vi "getParameters.vi"(8 "error in":errorcluster, 11 "Time in":refnum<class "Time.lvclass">) -> (0 "error out":errorcluster, 2 "Time.Parameters":T1, 3 "Time out":refnum<class "Time.lvclass">)   [LabVIEW 2022 SP3, in "Time.lvclass"]
uses:
  Time.lvclass
  Time.Parameters.ctl
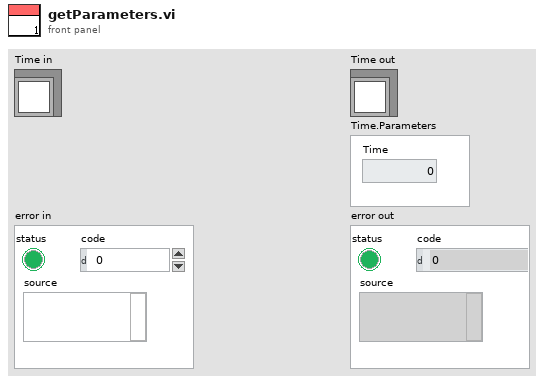
[diagram p1: front panel]
types:
  T1 = typedef "Time.lvclass/Time.Parameters.ctl" = cluster{"Time":u32}
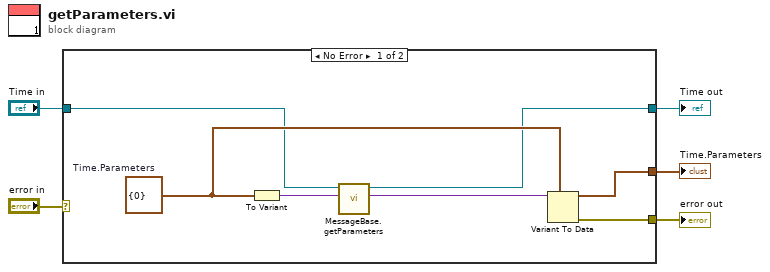
[diagram p0: block diagram]
diagram:
  n1 = case shown="No Error" "error in" {
    selector: "error in" -> [_ w14]
    tunnel: [w12 w14] -> w1
    tunnel: [w6 w13] -> w3
    tunnel: "Time in" -> [w8 w13]
    tunnel: [w11 _] -> w2
    frame No Error {
      w10 = T1 {"Time"=0}  # Time.Parameters
      n2 = To Variant(anything=w10) -> (Variant=w9:variant)
      n3 = call-dynamic "MessageBase.getParameters.vi"("Variant"=w9, "MessageBase in"=w8) -> ("Variant"=w7:variant, "MessageBase out"=w6:refnum<class "Time.lvclass">)  [unwired: 7 in, 1 out]
      n4 = Variant To Data(type=w10, Variant=w7) -> (data=w11:T1, error out=w12:errorcluster)  [unwired: 1 in]
    }
    frame Error {
    }
  }
  "error out" <- w1
  "Time out" <- w3
  "Time.Parameters" <- w2
